vi "Read INI File.vi"(8 "error in":errorcluster, 11 "Peer Review in":refnum<class "Peer Review.lvclass">) -> (0 "error out":errorcluster, 3 "Peer Review out":refnum<class "Peer Review.lvclass">)   [LabVIEW 2020, in "Peer Review.lvclass"]
uses:
  Peer Review.lvclass
  Peer Review.lvclass/Peer Review.ctl
  <vilib>/Utility/config.llb/Read Key (Path).vi
  <vilib>/Utility/config.llb/Read Key (Boolean).vi
  <vilib>/Utility/config.llb/Read Key (String).vi
  <vilib>/Utility/config.llb/NI_LVConfig.lvlib
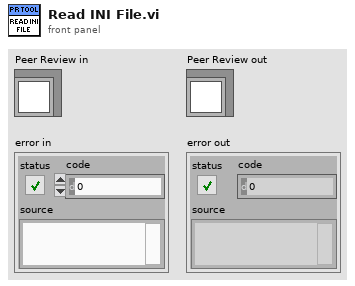
[diagram p1: front panel]
types:
  T1 = typedef "NI_LVConfig.lvlib/Config Data RefNum.ctl" = refnum<k1>
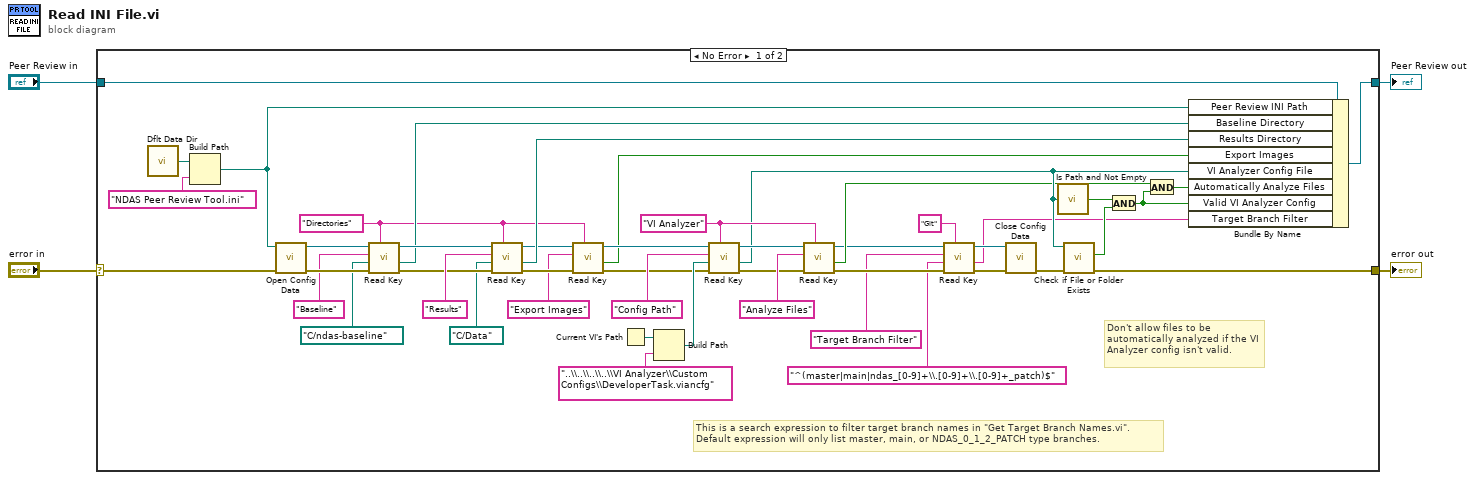
[diagram p0: block diagram]
diagram:
  n1 = case shown="No Error" "error in" {
    selector: "error in" -> [w44 w53]
    tunnel: [w28 w53] -> w3
    tunnel: "Peer Review in" -> [w30 w52]
    tunnel: [w40 w52] -> w1
    frame No Error {
      w31 = "VI Analyzer" ("section")
      w9 = "Directories" ("section")
      # "This is a search expression to filter target branch names in \"Get Target Branch Names.vi\".\nDefault expression will only list master, main, or NDAS_0_1_2_PATCH type branches."
      # "Don't allow files to be automatically analyzed if the VI Analyzer config isn't valid."
      n2 = call <vilib>:"Dflt Data Dir.vi"() -> ("App:Default Data Directory"=w20:path)
      n3 = Build Path(base path=w20, name or relative path="NDAS Peer Review Tool.ini") -> (appended path=w26:path)
      n4 = call <vilib>:"Open Config Data.vi"("error in (no error)"=w44, "configuration file path"=w26) -> ("error out"=w50:errorcluster, "refnum"=w49:T1)  [unwired: 7 in, 1 out]
      n5 = call-poly <vilib>:"Read Key.vi"("section"=w9, "error in (no error)"=w50, "default value"=path "C:/ndas-baseline" ("Baseline Directory"), "key"="Baseline" ("section"), "refnum"=w49) -> ("error out"=w45:errorcluster, "value"=w41:path, "refnum out"=w48:T1)  [unwired: 3 in, 1 out]
      n6 = call-poly <vilib>:"Read Key.vi"("section"=w9, "error in (no error)"=w45, "default value"=path "C:/Data" ("Results Directory"), "key"="Results" ("section"), "refnum"=w48) -> ("error out"=w10:errorcluster, "value"=w39:path, "refnum out"=w11:T1)  [unwired: 3 in, 1 out]
      n7 = call-poly <vilib>:"Read Key.vi"("section"=w9, "error in (no error)"=w10, "key"="Export Images" ("section"), "refnum"=w11) -> ("error out"=w7:errorcluster, "value"=w5:bool, "refnum out"=w6:T1)  [unwired: 4 in, 1 out]
      n8 = Current VI's Path() -> (path=w37:path)
      n9 = Build Path(base path=w37, name or relative path="..\\..\\..\\..\\VI Analyzer\\Custom Configs\\DeveloperTask.viancfg") -> (appended path=w32:path)
      n10 = call-poly <vilib>:"Read Key.vi"("section"=w31, "error in (no error)"=w7, "default value"=w32, "key"="Config Path" ("section"), "refnum"=w6) -> ("error out"=w35:errorcluster, "value"=w27:path, "refnum out"=w36:T1)  [unwired: 3 in, 1 out]
      n11 = call-poly <vilib>:"Read Key.vi"("section"=w31, "error in (no error)"=w35, "key"="Analyze Files", "refnum"=w36) -> ("error out"=w16:errorcluster, "value"=w23:bool, "refnum out"=w19:T1)  [unwired: 4 in, 1 out]
      n12 = call-poly <vilib>:"Read Key.vi"("section"="Git", "error in (no error)"=w16, "default value"="^(master|main|ndas_[0-9]+\\.[0-9]+\\.[0-9]+_patch)$", "key"="Target Branch Filter", "refnum"=w19) -> ("error out"=w17:errorcluster, "value"=w12:string, "refnum out"=w18:T1)  [unwired: 3 in, 1 out]
      n13 = call <vilib>:"Close Config Data.vi"("error in (no error)"=w17, "refnum"=w18) -> ("error out"=w29:errorcluster)  [unwired: 8 in, 1 out]
      n14 = call <vilib>:"Is Path and Not Empty.vi"("path"=w27) -> ("Is Path and Not Empty?"=w25:bool)  [unwired: 4 in]
      n15 = call <vilib>:"Check if File or Folder Exists.vi"("error in (no error)"=w29, "path"=w27) -> ("error out"=w28:errorcluster, "file or folder exists?"=w24:bool)  [unwired: 7 in, 1 out]
      n16 = And(x=w25, y=w24) -> (x .and. y?=w22:bool)
      n17 = And(x=w23, y=w22) -> (x .and. y?=w21:bool)
      n18 = Bundle By Name(cluster=w30, "Peer Review INI Path"=w26, "Baseline Directory"=w41, "Results Directory"=w39, "Export Images"=w5, "VI Analyzer Config File"=w27, "Automatically Analyze Files"=w21, "Valid VI Analyzer Config"=w22, "Target Branch Filter"=w12) -> (w40:refnum<class "Peer Review.lvclass">)
    }
    frame Error {
    }
  }
  "error out" <- w3
  "Peer Review out" <- w1
